vi "Get Desired Size.vi"(8 "error in (no error)":errorcluster, 11 "BoardArrayPanel in":refnum<class "BoardArrayPanel.lvclass">) -> (0 "error out":errorcluster, 2 "Desired Size":T1, 3 "BoardArrayPanel out":refnum<class "BoardArrayPanel.lvclass">)   [LabVIEW 2020, in "PicoG-App.lvlib" / "BoardArrayPanel.lvclass"]
uses:
  BoardArrayPanel.lvclass
  <vilib>/IlluminatedG/IG OOPanel/OOPanel/ArrayPanel/Desired Size.ctl
  <vilib>/IlluminatedG/IG OOPanel/OOPanel/OOPanel.lvlib
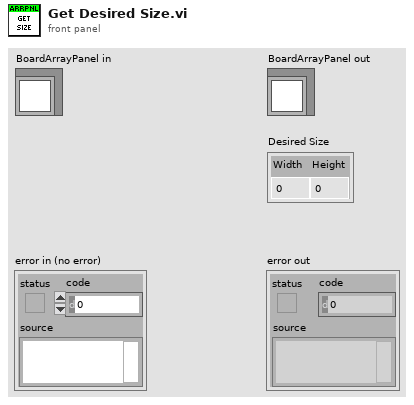
[diagram p1: front panel]
types:
  T1 = typedef "OOPanel.lvlib/Desired Size.ctl" = cluster{"Width":u32, "Height":u32}
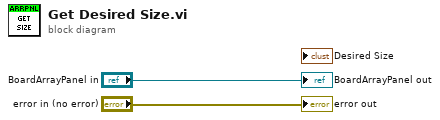
[diagram p0: block diagram]
diagram:
  "error out" <- "error in (no error)"
  "BoardArrayPanel out" <- "BoardArrayPanel in"
